vi "Mass Compile Directory for Current LV Version_COMPILE.vi"(6 "List only Top-Level files in llbs? (FALSE)":bool=TRUE, 8 "error in (no error)":errorcluster, 11 "Folder of LabVIEW files to convert":path) -> (0 "error out":errorcluster)   [LabVIEW 2023]
doc: "Mass compiles vi, vit, lvproj, and ctl files to a previous or current LabVIEW version. \n\nThe input path is traversed recursively. If the output path is left blank, the conveted files are saved in place."
uses:
  <userlib>/_OpenG.lib/file/file.llb/openg_file.lvlib
panel:
  out "Current File":path
  out "Converted files":path[](array[path])
  out "Array 2":errorcluster[](array[cluster])
  in  "Destination for converted files":path
  # "Mass Compile for current version"
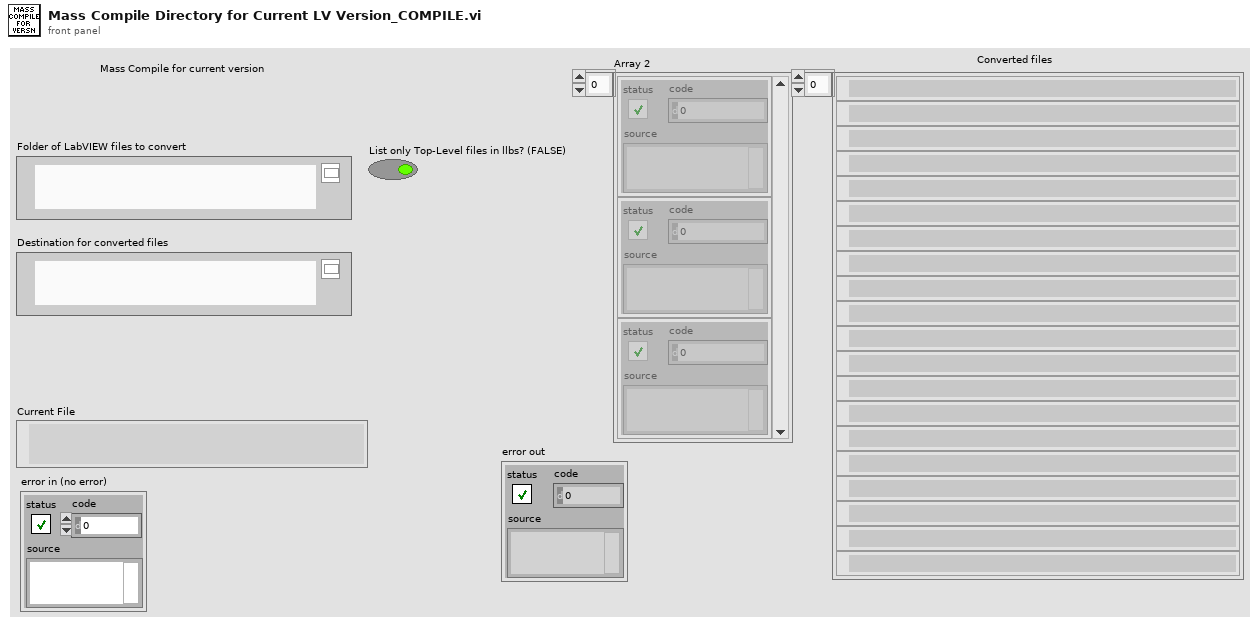
[diagram p1: front panel]
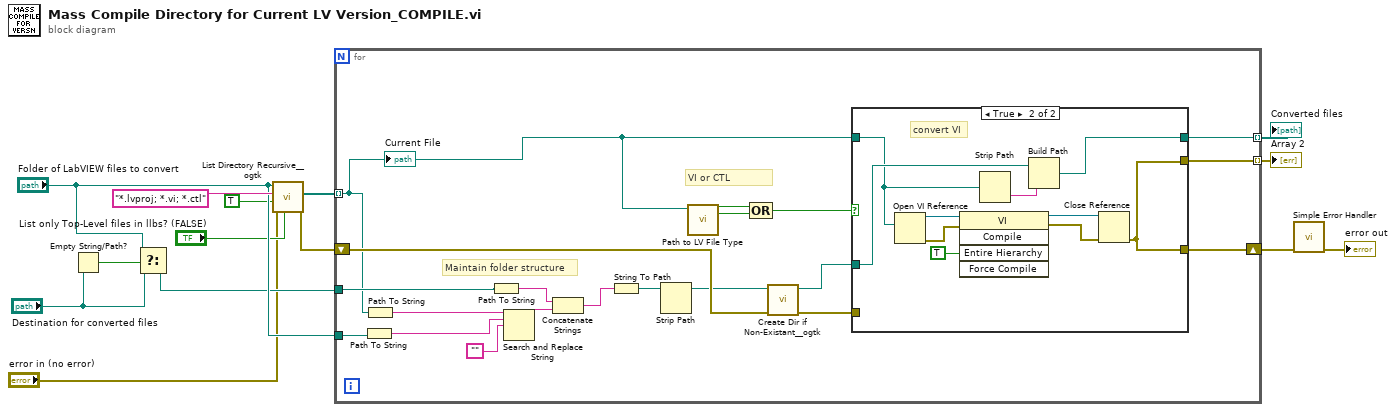
[diagram p0: block diagram]
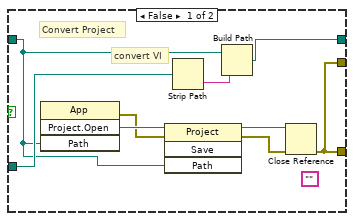
[diagram p2: hidden frame]
diagram:
  n1 = Empty String/Path?(string/path="Destination for converted files") -> (empty?=w8:bool)
  n2 = Select(t="Folder of LabVIEW files to convert", s=w8, f="Destination for converted files") -> (s? t:f=w5:path)
  n3 = call <userlib>:"List Directory Recursive__ogtk.vi"("List only Top-Level files in llbs? (FALSE)"="List only Top-Level files in llbs? (FALSE)", "error in (no error)"="error in (no error)", "Treat llb files as directories? (FALSE)"=TRUE, "pattern"="*.lvproj; *.vi; *.ctl", "Path"="Folder of LabVIEW files to convert") -> ("error out"=w12:errorcluster, "file paths"=w13:path[])  [unwired: 3 in, 2 out]
  n4 = for {
    shift-right: [w26] -> w14
    shift-left: w12 -> [w24]
    tunnel: w13 -> [w17] mode=indexing
    tunnel: w5 -> [w30]
    tunnel: "Folder of LabVIEW files to convert" -> [w34]
    tunnel: [w21] -> w10 mode=indexing
    tunnel: [w18] -> w9 mode=indexing
    # "VI or CTL"
    # "Maintain folder structure"
    n5 = Path To String(path=w34) -> (string=w32:string)
    n6 = Path To String(path=w17) -> (string=w33:string)
    n7 = Path To String(path=w30) -> (string=w29:string)
    n8 = Search and Replace String(input string=w33, search string=w32, replace string="") -> (result string=w28:string)  [unwired: 5 in, 3 out]
    n9 = Concatenate Strings(w29, w28) -> (w27:string)
    n10 = String To Path(string=w27) -> (path=w20:path)
    n11 = Strip Path(path=w20) -> (stripped path=w22:path)  [unwired: 1 out]
    n12 = call "Path to LV File Type.vi"("path"=w17) -> ("ctl"=w15:bool, "vi"=w16:bool)  [unwired: 5 in, 4 out]
    n13 = Compound Arithmetic op=OR(w16, w15) -> (w25:bool)
    n14 = call <userlib>:"Create Dir if Non-Existant__ogtk.vi"("error in (no error)"=w24, "Directory Path"=w22) -> ("error out"=w23:errorcluster, "dup Directory Path"=w19:path)  [unwired: 7 in, 1 out]
    n15 = case shown="True" w25 {
      tunnel: w19 -> [w38 w52]
      tunnel: [w39 w53] -> w26
      tunnel: w23 -> [_ _]
      tunnel: w17 -> [w35 w49]
      tunnel: [w39 w53] -> w21
      tunnel: [w36 w50] -> w18
      frame False {
        (unwired) ""
        # "convert VI"
        # "Convert Project"
        n16 = invoke class="App" method="Project.Open"("Path"=w35) -> (error out=w41:errorcluster, "Project:Open"=w43:refnum<vi>)  [unwired: 3 in, 2 out]
        n17 = invoke class="Project" method="Save"(reference=w43, error in=w41, "Path"=w35) -> (reference out=w42:refnum<vi>, error out=w40:errorcluster)  [unwired: 1 in, 2 out]
        n18 = Strip Path(path=w38) -> (name=w37:string)  [unwired: 1 out]
        n19 = Build Path(base path=w35, name or relative path=w37) -> (appended path=w36:path)
        n20 = Close Reference(reference=w42, error in (no error)=w40) -> (error out=w39:errorcluster)
      }
      frame True {
        # "convert VI"
        n21 = Open VI Reference(vi path=w49) -> (vi reference=w48:refnum<vi>, error out=w46:errorcluster)  [unwired: 5 in]
        n22 = invoke class="VI" method="Compile"(reference=w48, error in=w46, "Entire Hierarchy"=TRUE ("Compile Entire Hierarchy (F)")) -> (reference out=w47:refnum<vi>, error out=w45:errorcluster)  [unwired: 2 in, 3 out]
        n23 = Strip Path(path=w49) -> (name=w51:string)  [unwired: 1 out]
        n24 = Build Path(base path=w52, name or relative path=w51) -> (appended path=w50:path)
        n25 = Close Reference(reference=w47, error in (no error)=w45) -> (error out=w53:errorcluster)
      }
    }
    "Current File" <- w17
  }
  "Array 2" <- w10
  "Converted files" <- w9
  n26 = call <vilib>:"Simple Error Handler.vi"("error in (no error)"=w14) -> ("error out"=→"error out":errorcluster)  [unwired: 4 in, 4 out]
